vi "userDetailView.vi"() -> ()   [LabVIEW 2019]
doc: "40"
uses:
  03_Home/controller/logoutBtn.ctl
  03_Home/controller/exitBtn.ctl
  <vilib>/Utility/miscctls.llb/LVPointTypeDef.ctl
  03_Home/controller/pannelState.ctl
  globalValue.vi
panel:
  in  "backPage":bool
  out "user_id":string
  out "userDetailInfo":string[](array[string])
  in  "passwordResetBtn":bool
  in  "updateBtn":bool
  in  "deleteBtn":bool
  in  "role":string(combo)
  in  "securityQuestion":string(combo)
  in  "securityAnswer":string
  in  "userEmail":string
  in  "userPhone":string
  in  "userNm":string
  out "userLoginId":string
  in  "Help Button":bool
  in  "LogOut Button":T1
  in  "Exit Button":T2
  out "userNm":string
  # "|"
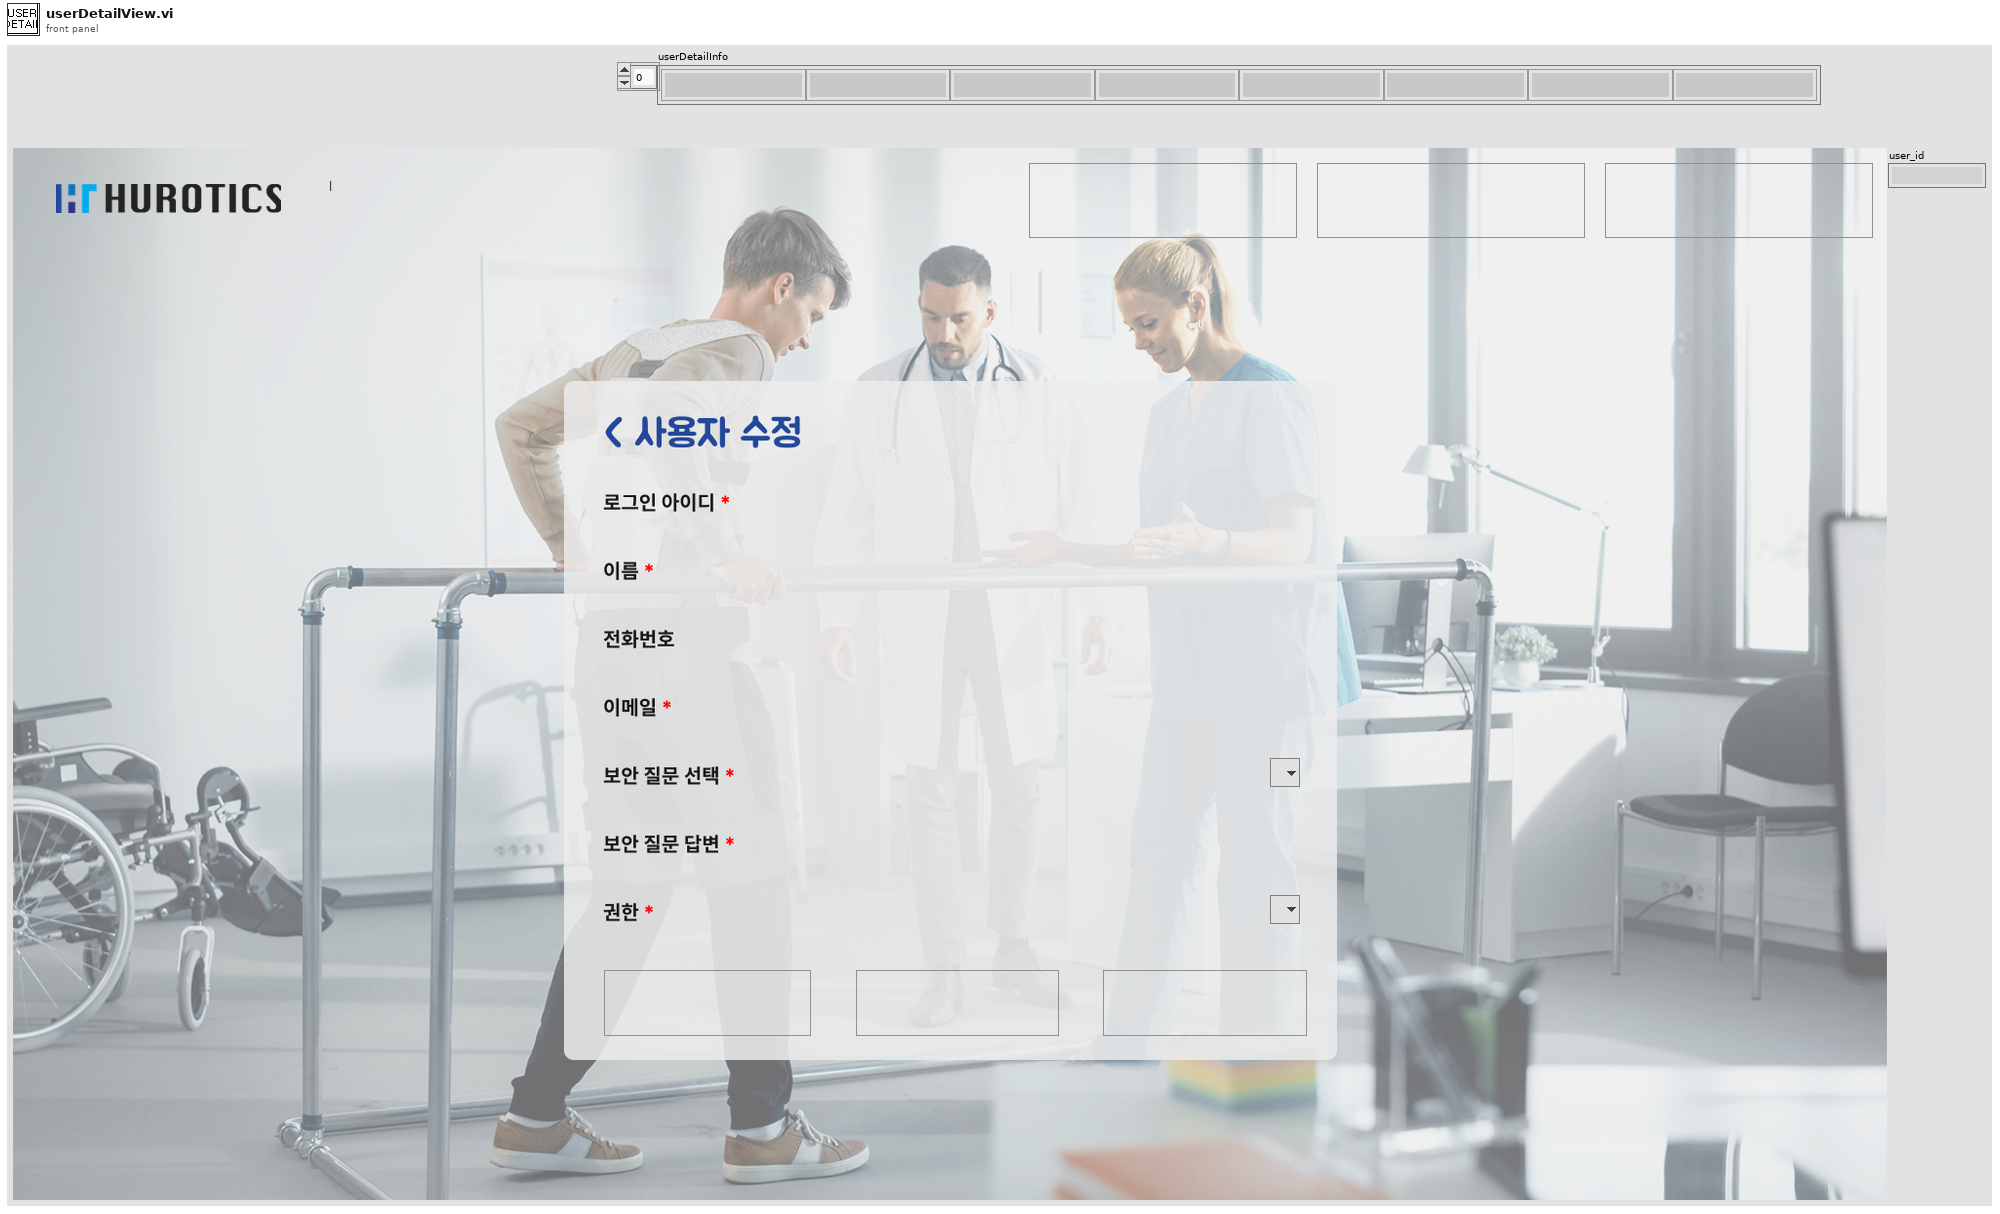
[diagram p1: front panel]
types:
  T1 = typedef "logoutBtn.ctl" = bool
  T2 = typedef "exitBtn.ctl" = bool
  T3 = typedef "LVPointTypeDef.ctl" = cluster{"Horizontal":i16, "Vertical":i16}
  T4 = enum16{"connection", "create", "getReadList", "getRead", "getCount", "update", "delete", "close"}
  T5 = typedef "pannelState.ctl" = enum16{"Init", "LogIn", "SignUpView", "Home", "Management_patientList", "Management_patientTrashtList", "Management_patientCreate", "Management_patientUpdate", "Management_patientTraining", "Management_patientTrainingDetail", "H-MEDI PatientList", "H-MEDI HardwareCtl", "Adjust", "FineTuning", "UserList", "UserDetail", "Exit"}
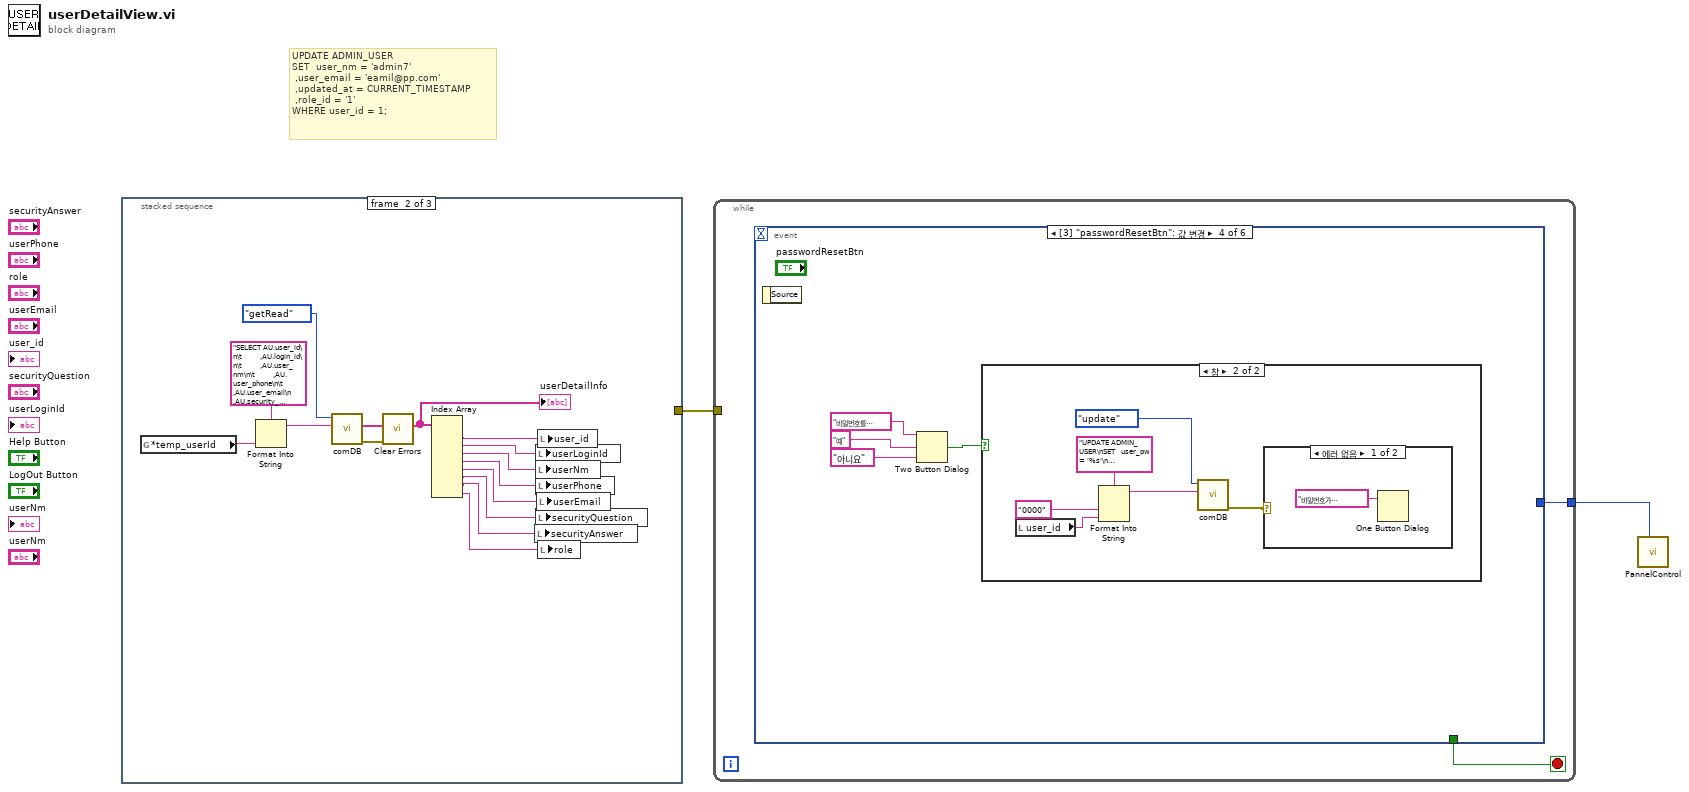
[diagram p0: block diagram]
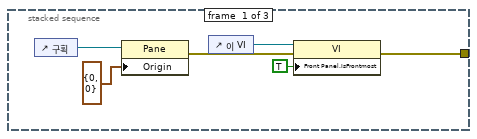
[diagram p2: hidden frame]
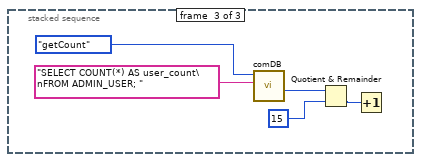
[diagram p3: hidden frame]
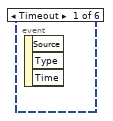
[diagram p4: hidden frame]
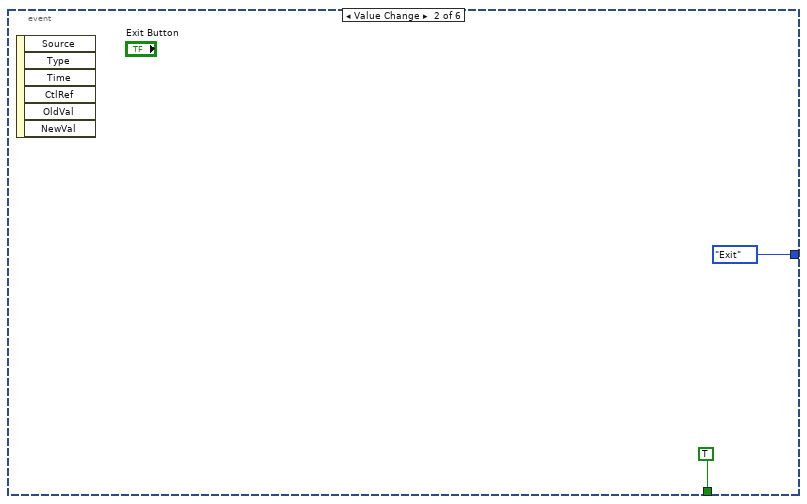
[diagram p5: hidden frame]
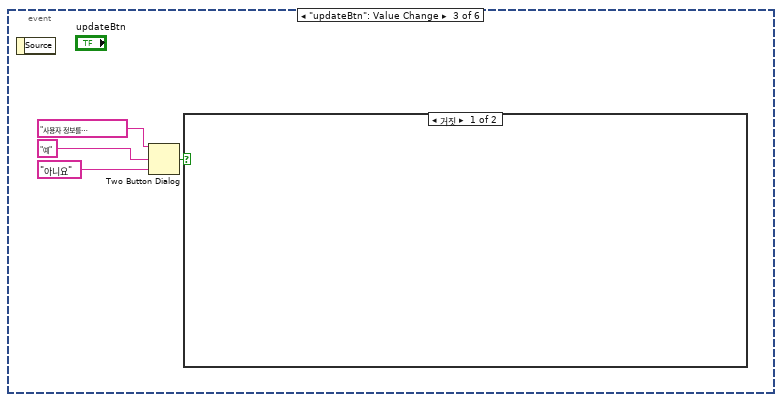
[diagram p6: hidden frame]
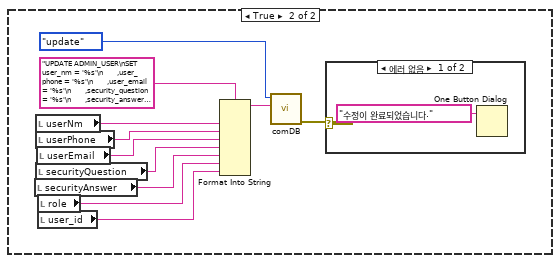
[diagram p7: hidden frame]
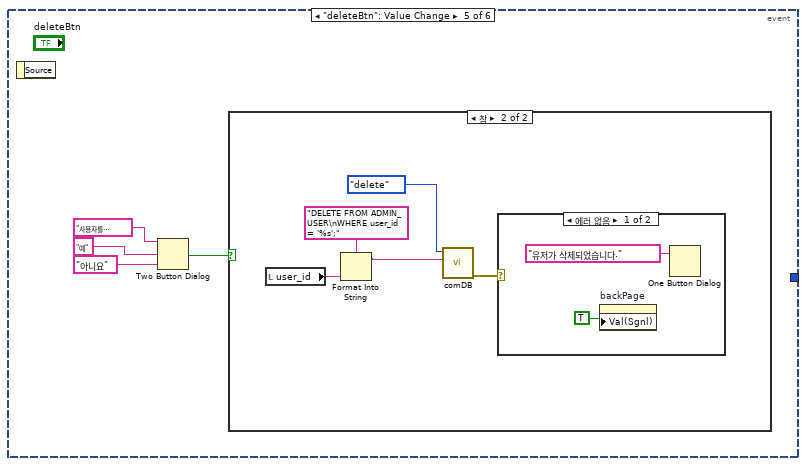
[diagram p11: hidden frame]
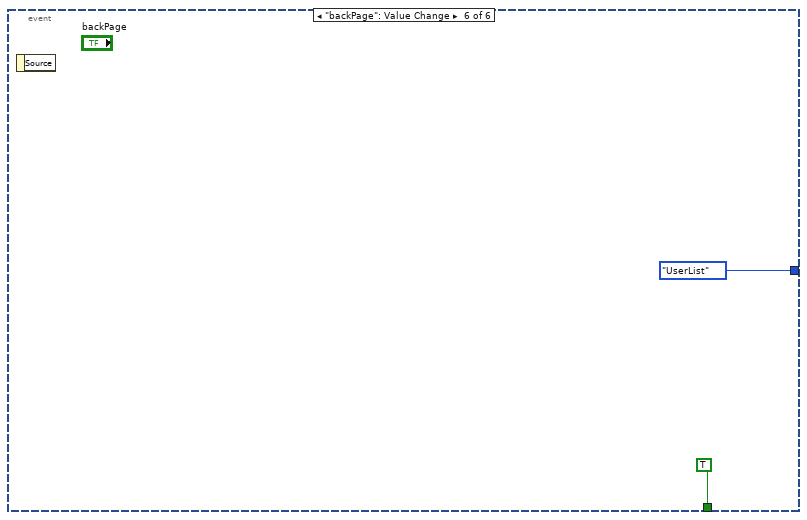
[diagram p14: hidden frame]
diagram:
  # "UPDATE ADMIN_USER\nSET  user_nm = 'admin7'\n\t,user_email = 'eamil@pp.com'\n\t,updated_at = CURRENT_TIMESTAMP\n\t,role_id = '1'\nWHERE user_id = 1;"
  n1 = stacked-sequence {
    tunnel: [w3 _ _] -> w1
    frame #0 {
      n2 = control-ref of="구획"() -> (w6:refnum<vi>)
      n3 = property class="Pane"(reference=w6, "Origin"=T3 {"Horizontal"=0, "Vertical"=0} ("원점")) -> (error out=w4:errorcluster)  [unwired: 1 in, 1 out]
      n4 = control-ref of="이 VI"() -> (w8:refnum<vi>)
      n5 = property class="VI"(reference=w8, error in=w4, "Front Panel.IsFrontmost"=TRUE ("프런트패널 윈도우:맨 앞으로")) -> (error out=w3:errorcluster)  [unwired: 1 out]
    }
    frame #1 {
      n6 = global read "globalValue.vi" "*temp_userId"() -> (w9:string)
      n7 = Format Into String(format string="SELECT AU.user_id\n\t         ,AU.login_id\n\t         ,AU.user_nm\n\t         ,AU.user_phone\n\t         ,AU.user_email\n          ,AU.security_question\n          ,AU.security_answer\n          ,R.role_id\n          ,R.role_nm\nFROM ADMIN_USER AU\nJOIN ROLE R ON AU.role_id = R.role_id\nWHERE AU.user_id = '%s'" ("Query"), w9) -> (resulting string=w21:string)  [unwired: 2 in, 1 out]
      n8 = call "comDB.vi"("Query"=w21, "State"=T4."getRead") -> ("error out"=w10:errorcluster, "result1DArray"=w19:string[])  [unwired: 5 in, 2 out]
      "userDetailInfo" <- w19
      n9 = call <vilib>:"Clear Errors.vi"("error in (no error)"=w10) -> ()  [unwired: 5 in, 2 out]
      n10 = Index Array(array=w19) -> (element #1=w11:string, element #2=w18:string, element #3=w17:string, element #4=w16:string, element #5=w15:string, element #6=w14:string, element #7=w13:string, element #8=w12:string)  [unwired: 8 in]
      n11 = local write "securityAnswer"(w13) -> ()
      n12 = local write "userLoginId"(w18) -> ()
      n13 = local write "userNm"(w17) -> ()
      n14 = local write "userPhone"(w16) -> ()
      n15 = local write "securityQuestion"(w14) -> ()
      n16 = local write "userEmail"(w15) -> ()
      n17 = local write "user_id"(w11) -> ()
      n18 = local write "role"(w12) -> ()
    }
    frame #2 {
      n19 = call "comDB.vi"("Query"="SELECT COUNT(*) AS user_count\nFROM ADMIN_USER; ", "State"=T4."getCount") -> ("count"=w23:i64)  [unwired: 5 in, 3 out]
      n20 = Quotient & Remainder(x=w23, y=i64 15) -> (floor(x/y)=w24:i64)  [unwired: 1 out]
      n21 = Increment(x=w24) -> ()  [unwired: 1 out]
    }
  }
  n22 = while {
    tunnel: [w28] -> w2
    tunnel: w1 -> [_]
    stop <- w29 stop-if-true
    n23 = event shown="[3] \"passwordResetBtn\": 값 변경" {
      selector: _ -> [_ _ _ _ _ _]
      dyn-events: _ -> [_ _ _ _ _ _]
      timeout: _ -> [_ _ _ _ _ _]
      tunnel: [_ TRUE _ _ _ TRUE] -> w29
      tunnel: [_ pannelState."Exit" ("State") _ _ _ pannelState."UserList" ("State")] -> w28
      event Timeout {
        n24 = event-data() -> ()  [unwired: 1 in, 3 out]
      }
      event Value Change {
        n25 = event-data() -> ()  [unwired: 1 in, 6 out]
      }
      event "updateBtn": Value Change {
        n26 = event-data() -> ()  [unwired: 1 in, 1 out]
        n27 = Two Button Dialog(message="사용자 정보를 수정하시겠습니까?" ("메시지"), 1:"아니요" ("거짓 버튼 이름(\"취소\")"), 2:"예" ("참 버튼 이름(\"확인\")")) -> (T button?=w32:bool)
        n28 = case shown="거짓" w32 {
          frame False {
          }
          frame True {
            n29 = local read "securityAnswer"() -> (w41:string)
            n30 = local read "userNm"() -> (w45:string)
            n31 = local read "userPhone"() -> (w44:string)
            n32 = local read "securityQuestion"() -> (w42:string)
            n33 = local read "userEmail"() -> (w43:string)
            n34 = local read "role"() -> (w40:string)
            n35 = local read "user_id"() -> (w39:string)
            n36 = Format Into String(format string="UPDATE ADMIN_USER\nSET   user_nm = '%s'\n       ,user_phone = '%s'\n       ,user_email = '%s'\n       ,security_question = '%s'\n       ,security_answer = '%s'\n       ,role_id = '%s'\n       ,updated_at = CURRENT_TIMESTAMP\nWHERE user_id = '%s'" ("Query"), w45, w44, w43, w42, w41, w40, w39) -> (resulting string=w37:string)  [unwired: 2 in, 1 out]
            n37 = call "comDB.vi"("Query"=w37, "State"=T4."update") -> ("error out"=w36:errorcluster)  [unwired: 5 in, 3 out]
            n38 = case shown="에러 없음" w36 {
              frame No Error {
                n39 = One Button Dialog(message="수정이 완료되었습니다." ("메시지")) -> ()  [unwired: 1 in, 1 out]
              }
              frame Error {
              }
            }
          }
        }
      }
      event "passwordResetBtn": Value Change {
        n40 = event-data() -> ()  [unwired: 1 in, 1 out]
        n41 = Two Button Dialog(message="비밀번호를 '0000'으로 초기화하시겠습니까?" ("메시지"), 1:"아니요" ("거짓 버튼 이름(\"취소\")"), 2:"예" ("참 버튼 이름(\"확인\")")) -> (T button?=w48:bool)
        n42 = case shown="참" w48 {
          frame False {
          }
          frame True {
            n43 = local read "user_id"() -> (w56:string)
            n44 = Format Into String(format string="UPDATE ADMIN_USER\nSET   user_pw = '%s'\n       ,updated_at = CURRENT_TIMESTAMP\nWHERE user_id = '%s'" ("Query"), "0000", w56) -> (resulting string=w54:string)  [unwired: 2 in, 1 out]
            n45 = call "comDB.vi"("Query"=w54, "State"=T4."update") -> ("error out"=w53:errorcluster)  [unwired: 5 in, 3 out]
            n46 = case shown="에러 없음" w53 {
              frame No Error {
                n47 = One Button Dialog(message="비밀번호가 초기화되었습니다." ("메시지")) -> ()  [unwired: 1 in, 1 out]
              }
              frame Error {
              }
            }
          }
        }
      }
      event "deleteBtn": Value Change {
        n48 = event-data() -> ()  [unwired: 1 in, 1 out]
        n49 = Two Button Dialog(message="사용자를 삭제하시겠습니까?" ("메시지"), 1:"아니요" ("거짓 버튼 이름(\"취소\")"), 2:"예" ("참 버튼 이름(\"확인\")")) -> (T button?=w59:bool)
        n50 = case shown="참" w59 {
          frame False {
          }
          frame True {
            n51 = local read "user_id"() -> (w63:string)
            n52 = Format Into String(format string="DELETE FROM ADMIN_USER\nWHERE user_id = '%s';" ("Query"), w63) -> (resulting string=w65:string)  [unwired: 2 in, 1 out]
            n53 = call "comDB.vi"("Query"=w65, "State"=T4."delete") -> ("error out"=w64:errorcluster)  [unwired: 5 in, 3 out]
            n54 = case shown="에러 없음" w64 {
              frame No Error {
                n55 = property on="backPage" class="Bool (엄격한)"("Val(Sgnl)"=TRUE ("backPage")) -> ()  [unwired: 2 in, 2 out]
                n56 = One Button Dialog(message="유저가 삭제되었습니다." ("메시지")) -> ()  [unwired: 1 in, 1 out]
              }
              frame Error {
              }
            }
          }
        }
      }
      event "backPage": Value Change {
        n57 = event-data() -> ()  [unwired: 1 in, 1 out]
      }
    }
  }
  n58 = call "PannelControl.vi"("State"=w2) -> ()  [unwired: 10 in, 1 out]
